vi "Execute Shortcut Menu Selection.vi"(8 "Error In":errorcluster, 9 "Tree Tag":string, 10 "Menu Tag":string, 11 "Bookmarks":T1[](array[typedef])) -> (0 "Error Out":errorcluster)   [LabVIEW 2017, in "Bookmark Manager.lvlib"]
uses:
  Bookmark Manager.lvlib
  Controls/VI Bookmark.ctl
  Controls/VI Information.ctl
  Controls/Application Information.ctl
  Toolkit VIs/Toolkit.lvlib
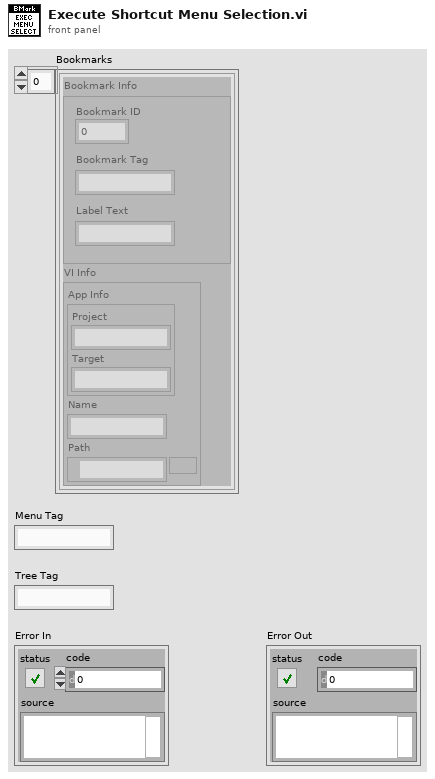
[diagram p1: front panel]
types:
  T1 = typedef "Bookmark Manager.lvlib/VI Bookmark.ctl" = cluster{"Bookmark Info":cluster{"Bookmark ID":u32, "Bookmark Tag":string, "Label Text":string}, "VI Info":T2}
  T2 = typedef "Bookmark Manager.lvlib/VI Information.ctl" = cluster{"App Info":T3, "Name":string, "Path":path}
  T3 = typedef "Bookmark Manager.lvlib/Application Information.ctl" = cluster{"Project":string, "Target":string}
  T4 = enum32{"Bad", "Idle", "Run top level", "Running"}
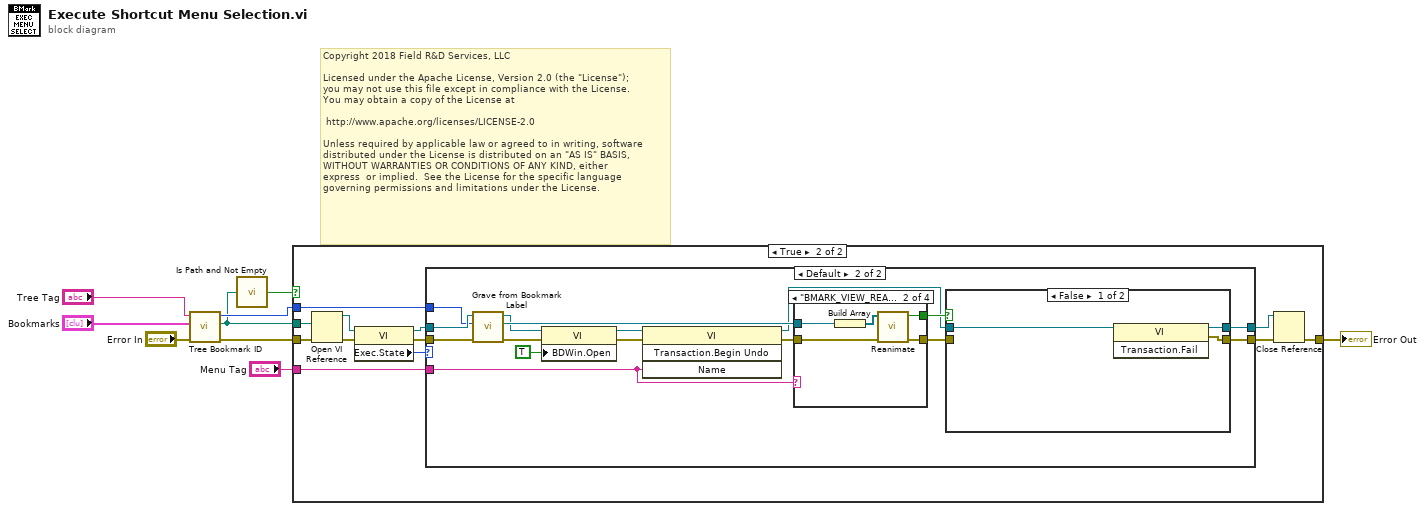
[diagram p0: block diagram]
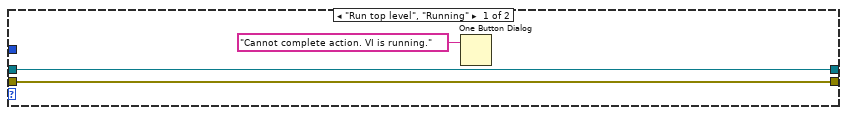
[diagram p3: hidden frame]
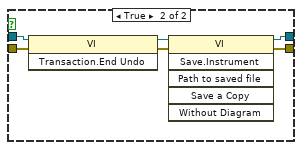
[diagram p4: hidden frame]
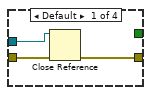
[diagram p5: hidden frame]
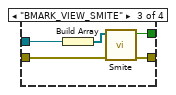
[diagram p6: hidden frame]
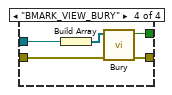
[diagram p7: hidden frame]
diagram:
  # "Copyright 2018 Field R&D Services, LLC\n\nLicensed under the Apache License, Version 2.0 (the \"License\");\nyou may not use this file except in compliance with the License.\nYou may obtain a copy of the License at\n\n\thttp://www.apache.org/licenses/LICENSE-2.0\n\nUnless required by applicable law or agreed to in writing, software\ndistributed under the License is distributed on an \"AS IS\" BASIS,\nWITHOUT WARRANTIES OR CONDITIONS OF ANY KIND, either \nexpress  or implied.  See the License for the specific language \ngoverning permissions and limitations under the License."
  n1 = call "Tree Bookmark ID.vi"("Error In"="Error In", "Bookmarks"="Bookmarks", "Tag"="Tree Tag") -> ("Error Out"=w1:errorcluster, "Path"=w4:path, "Bookmark ID"=w5:u32)  [unwired: 6 in]
  n2 = call <vilib>:"Is Path and Not Empty.vi"("path"=w4) -> ("Is Path and Not Empty?"=w3:bool)  [unwired: 4 in]
  n3 = case shown="True" w3 {
    tunnel: [w10 w22] -> w7
    tunnel: "Menu Tag" -> [_ w16]
    tunnel: w4 -> [_ w13]
    tunnel: w5 -> [_ w12]
    tunnel: w1 -> [w10 w11]
    frame False {
    }
    frame True {
      n4 = Open VI Reference(vi path=w13, error in (no error)=w11) -> (vi reference=w15:refnum<vi>, error out=w14:errorcluster)  [unwired: 4 in]
      n5 = property class="VI"(reference=w15, error in=w14) -> (reference out=w19:refnum<vi>, error out=w20:errorcluster, "Exec.State"=w21:T4)
      n6 = case shown="Default" w21 {
        tunnel: [w24 w31] -> w17
        tunnel: w20 -> [w24 w41]
        tunnel: w19 -> [w25 w39]
        tunnel: [w25 w32] -> w18
        tunnel: w16 -> [_ w26]
        tunnel: w12 -> [_ w37]
        frame "Run top level", "Running" {
          n7 = One Button Dialog(message="Cannot complete action. VI is running.") -> ()  [unwired: 1 in, 1 out]
        }
        frame Default {
          n8 = call "Grave from Bookmark Label.vi"("Error In"=w41, "Bookmark ID"=w37, "VI In"=w39) -> ("Error Out"=w35:errorcluster, "Grave"=w40:refnum<vi>, "VI Out"=w38:refnum<vi>)  [unwired: 6 in]
          n9 = property class="VI"(reference=w38, error in=w35, "BDWin.Open"=TRUE ("Block Diagram Window:Open")) -> (reference out=w36:refnum<vi>, error out=w34:errorcluster)
          n10 = invoke class="VI" method="Transaction.Begin Undo"(reference=w36, error in=w34, "Name"=w26) -> (reference out=w28:refnum<vi>, error out=w27:errorcluster)  [unwired: 1 in, 2 out]
          n11 = case shown="\"BMARK_VIEW_REANIMATE\"" w26 {
            tunnel: w40 -> [w53 w58 w63 w68]
            tunnel: [w51 w56 w60 w66] -> w30
            tunnel: [_ w55 w59 w65] -> w29
            tunnel: w27 -> [w52 w54 w61 w64]
            frame Default {
              n12 = Close Reference(reference=w53, error in (no error)=w52) -> (error out=w51:errorcluster)
            }
            frame "BMARK_VIEW_REANIMATE" {
              n13 = Build Array(w58) -> (w57:refnum<vi>[])
              n14 = call "Reanimate.vi"("Error In"=w54, "Graves"=w57) -> ("Error Out"=w56:errorcluster, "Change Made?"=w55:bool)  [unwired: 8 in]
            }
            frame "BMARK_VIEW_SMITE" {
              n15 = Build Array(w63) -> (w62:refnum<vi>[])
              n16 = call "Smite.vi"("Error In"=w61, "Graves"=w62) -> ("Error Out"=w60:errorcluster, "Change Made?"=w59:bool)  [unwired: 8 in]
            }
            frame "BMARK_VIEW_BURY" {
              n17 = Build Array(w68) -> (w67:refnum<vi>[])
              n18 = call "Bury.vi"("Error In"=w64, "Graves"=w67) -> ("Error Out"=w66:errorcluster, "Change Made?"=w65:bool)  [unwired: 8 in]
            }
          }
          n19 = case shown="False" w29 {
            tunnel: [w44 w49] -> w32
            tunnel: [w43 w47] -> w31
            tunnel: w30 -> [_ w46]
            tunnel: w28 -> [w42 w45]
            frame False {
              n20 = invoke class="VI" method="Transaction.Fail"(reference=w42) -> (reference out=w44:refnum<vi>, error out=w43:errorcluster)  [unwired: 2 in, 1 out]
            }
            frame True {
              n21 = invoke class="VI" method="Transaction.End Undo"(reference=w45, error in=w46) -> (reference out=w50:refnum<vi>, error out=w48:errorcluster)  [unwired: 1 in, 1 out]
              n22 = invoke class="VI" method="Save.Instrument"(reference=w50, error in=w48) -> (reference out=w49:refnum<vi>, error out=w47:errorcluster)  [unwired: 4 in, 4 out]
            }
          }
        }
      }
      n23 = Close Reference(reference=w18, error in (no error)=w17) -> (error out=w22:errorcluster)
    }
  }
  "Error Out" <- w7
